vi "Parse U32 Ind Regs.vi"(10 "ECUEvents In":T2, 11 "U32 Registers":T3[](array[typedef])) -> (2 "ECUEvents Out":T2)   [LabVIEW 2011, in "Engine Sim System Explorer.lvlib"]
uses:
  Engine Sim System Explorer.lvlib
  <userlib>/_FPGA Interface Advanced Tools/FPGA Bitfile Utility/TypeDefs/Scalar Register.ctl
  TypeDefs/ECUEventRegs.ctl
  <userlib>/_FPGA Interface Advanced Tools/FPGA Bitfile Utility/FPGA Bitfile Utility.lvlib
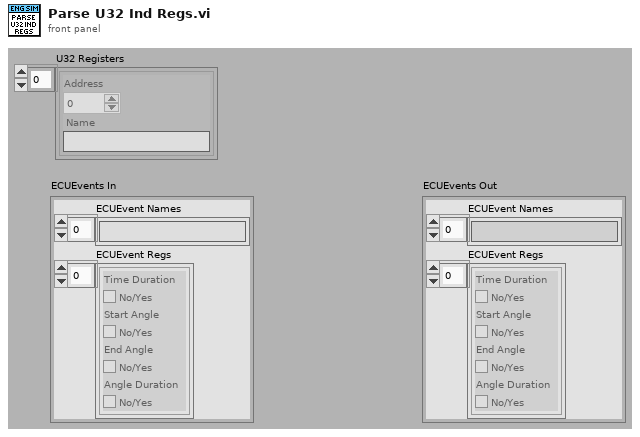
[diagram p1: front panel]
types:
  T1 = typedef "Engine Sim System Explorer.lvlib/ECUEventRegs.ctl" = cluster{"Time Duration":bool, "Start Angle":bool, "End Angle":bool, "Angle Duration":bool}
  T2 = cluster{"ECUEvent Names":string[], "ECUEvent Regs":T1[]}
  T3 = typedef "FPGA Bitfile Utility.lvlib/Scalar Register.ctl" = cluster{"Address":u32, "Name":string}
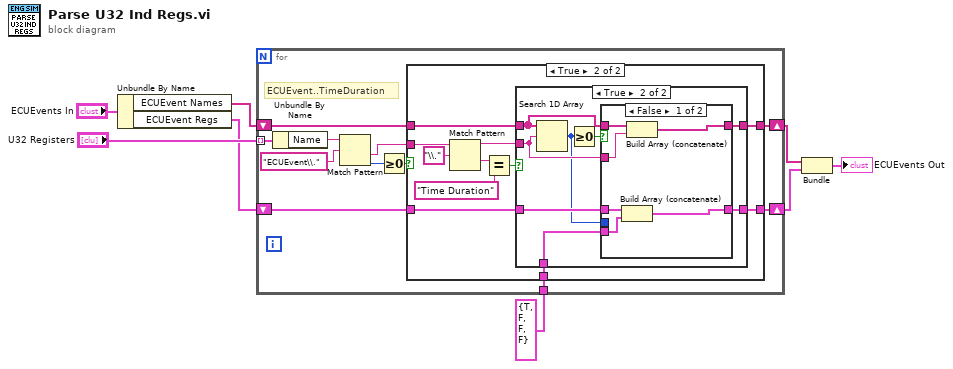
[diagram p0: block diagram]
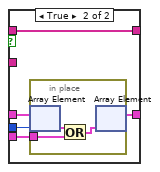
[diagram p4: hidden frame]
diagram:
  n1 = Unbundle By Name("ECUEvents In") -> ("ECUEvent Names"=w5:string[], "ECUEvent Regs"=w4:T1[])
  n2 = for {
    tunnel: "U32 Registers" -> [w19] mode=indexing
    tunnel: T1 {"Time Duration"=TRUE, "Start Angle"=FALSE, "End Angle"=FALSE, "Angle Duration"=FALSE} ("ECUEvent Registers") -> [w13]
    shift-right: [w12] -> w2
    shift-left: w4 -> [w11]
    shift-right: [w10] -> w3
    shift-left: w5 -> [w9]
    # "ECUEvent..TimeDuration"
    n3 = Unbundle By Name(w19) -> ("Name"=w18:string)
    n4 = Match Pattern(string=w18, regular expression="ECUEvent\\.") -> (after substring=w14:string, offset past match=w16:i32)  [unwired: 1 in, 2 out]
    n5 = Greater Or Equal To 0?(x=w16) -> (x >= 0?=w15:bool)
    n6 = case shown="True" w15 {
      tunnel: w14 -> [_ w32]
      tunnel: w13 -> [_ w24]
      tunnel: [w20 w22] -> w12
      tunnel: w11 -> [w20 w26]
      tunnel: [w21 w23] -> w10
      tunnel: w9 -> [w21 w28]
      frame False {
      }
      frame True {
        n7 = Match Pattern(string=w32, regular expression="\\.") -> (before substring=w27:string, after substring=w30:string)  [unwired: 1 in, 2 out]
        n8 = Equal?(x=w30, y="Time Duration") -> (x = y?=w25:bool)
        n9 = case shown="True" w25 {
          tunnel: w27 -> [_ w37]
          tunnel: w24 -> [_ w40]
          tunnel: [w33 w39] -> w22
          tunnel: w26 -> [w33 w41]
          tunnel: [w34 w36] -> w23
          tunnel: w28 -> [w34 w38]
          frame False {
          }
          frame True {
            n10 = Search 1D Array(1D array=w38, element=w37) -> (index of element=w35:i32)  [unwired: 1 in]
            n11 = Greater Or Equal To 0?(x=w35) -> (x >= 0?=w42:bool)
            n12 = case shown="False" w42 {
              tunnel: w41 -> [w48 w52]
              tunnel: w40 -> [w47 w50]
              tunnel: [w46 w49] -> w39
              tunnel: w38 -> [w45 w53]
              tunnel: w37 -> [w44 _]
              tunnel: [w43 w53] -> w36
              tunnel: w35 -> [_ w51]
              frame False {
                n13 = Build Array (concatenate)(w48, w47) -> (w46:T1[])
                n14 = Build Array (concatenate)(w45, w44) -> (w43:string[])
              }
              frame True {
                n15 = in-place {
                  in-place-border: w50 -> [w55]
                  n16 = in-place-array #1(w52, w51) -> (w56:T1)
                  n17 = Or(x=w56, y=w55) -> (x .or. y?=w54:T1)
                  n18 = in-place-array #1(w54) -> (w49:T1[])  [unwired: 1 out]
                }
              }
            }
          }
        }
      }
    }
  }
  n19 = Bundle("ECUEvent Names"=w3, "ECUEvent Regs"=w2) -> (→"ECUEvents Out":T2)  [unwired: 1 in]
